vi "disgardComPort.vi"(2 "error in (no error)":errorcluster, 3 "BK1823ACounter.lvclass":refnum<class "BK1823ACounter.lvclass">) -> (0 "error out":errorcluster, 1 "BK1823ACounter.lvclass 2":refnum<class "BK1823ACounter.lvclass">)   [LabVIEW 2009, in "Hardware.lvlib" / "frequencyCounters.lvlib" / "BK1823ACounter.lvclass"]
uses:
  BK1823ACounter.lvclass
  BK1823ACounter.lvclass/BK1823ACounter.ctl
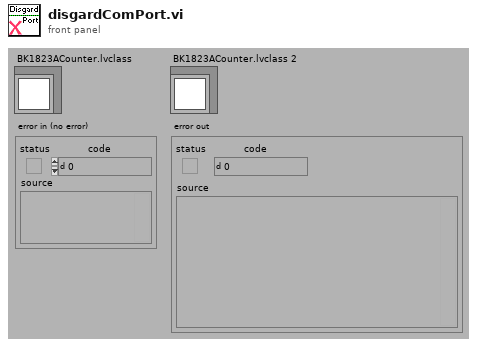
[diagram p1: front panel]
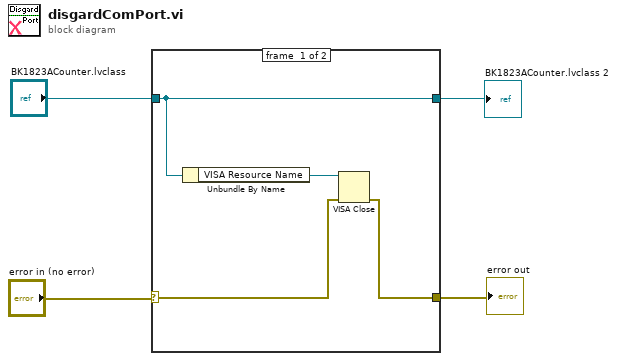
[diagram p0: block diagram]
diagram:
  n1 = case shown="No Error" "error in (no error)" {
    selector: "error in (no error)" -> [w8 w10]
    tunnel: [w7 w10] -> w3
    tunnel: "BK1823ACounter.lvclass" -> [w5 w9]
    tunnel: [w5 w9] -> w1
    frame #0 {
      n2 = Unbundle By Name(w5) -> ("VISA Resource Name"=w6:refnum<visa-resource-name>)
      n3 = VISA Close(VISA resource name=w6, error in (no error)=w8) -> (error out=w7:errorcluster)
    }
    frame #1 {
    }
  }
  "error out" <- w3
  "BK1823ACounter.lvclass 2" <- w1
